vi "Word Search.vi"(8 "error in (no error)":errorcluster, 9 "Solver VI":T1, 10 "Word List":string[](array[string])=["YELLOW", "ORANGE", "PURPLE", "BLUE", "GREEN", "RED"], 11 "Word Search Grid":string[][](array[string])=[["R", "B", "L", "U", "E", "W"], ["E", "G", "N", "A", "R", "O"], ["D", "B", "C", "E", "W", "L"], ["L", "L", "D", "K", "V", "L"], ["P", "U", "R", "P", "L", "E"], ["N", "E", "E", "R", "G", "Y"]]) -> (0 "error out":errorcluster, 2 "All Words Found":bool, 3 "Execution Time":dbl)   [LabVIEW 2024, in "Wordle Scorer.lvlib"]
uses:
  Wordle Scorer.lvlib
  Solver VI Ref Type.ctl
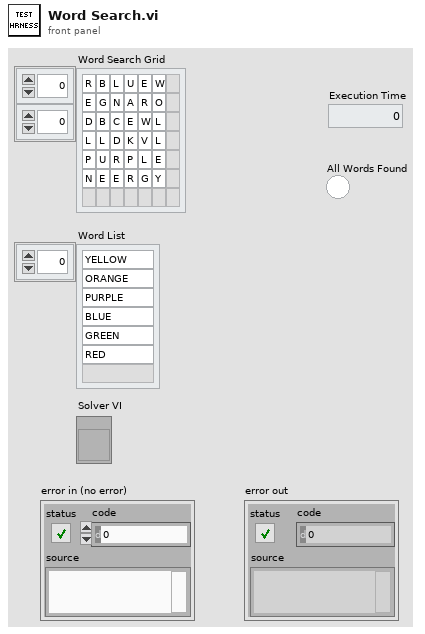
[diagram p1: front panel]
types:
  T1 = typedef "Wordle Scorer.lvlib/Solver VI Ref Type.ctl" = refnum<vi>
  T2 = typedef "Word Search Scorer.lvlib/Solutions--map.ctl" = map{string, T3[]}
  T3 = typedef "Word Search Scorer.lvlib/Letter Index--cluster.ctl" = cluster{"Row":i32, "Column":i32}
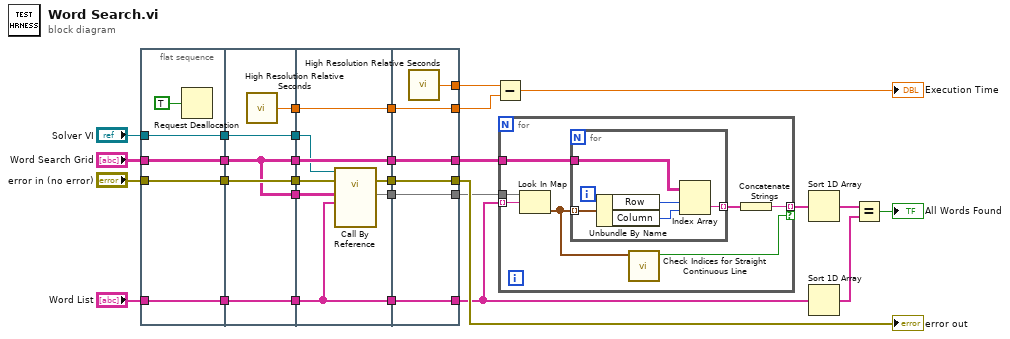
[diagram p0: block diagram]
diagram:
  n1 = flat-sequence {
    tunnel: "error in (no error)" -> [w32]
    tunnel: "Solver VI" -> [w33]
    tunnel: "Word List" -> [w34]
    tunnel: "Word Search Grid" -> [w35]
    tunnel: [w35] -> w4
    tunnel: [w34] -> w3
    tunnel: [w33] -> w2
    tunnel: [w32] -> w1
    tunnel: [w39] -> w29
    tunnel: [w37] -> w28
    tunnel: [w38] -> w26
    tunnel: [w37] -> w22
    tunnel: [w36] -> w21
    tunnel: [w40] -> w7
    tunnel: w4 -> [w37]
    tunnel: w3 -> [w39]
    tunnel: w2 -> [w36]
    tunnel: w1 -> [w40]
    tunnel: w29 -> [w44]
    tunnel: w28 -> [w45]
    tunnel: [w43] -> w27
    tunnel: w26 -> [w48]
    tunnel: [w48] -> w25
    tunnel: [w44] -> w24
    tunnel: [w47] -> w23
    tunnel: w22 -> [w47]
    tunnel: w21 -> [w46]
    tunnel: w7 -> [w42]
    tunnel: [w41] -> w5
    tunnel: w27 -> [w51]
    tunnel: w25 -> [w53]
    tunnel: w24 -> [w50]
    tunnel: w23 -> [w52]
    tunnel: [w54] -> w12
    tunnel: [w53] -> w11
    tunnel: [w52] -> w8
    tunnel: [w51] -> w10
    tunnel: [w50] -> w9
    tunnel: [w49] -> w30
    tunnel: w5 -> [w49]
    frame #0 {
      n2 = Request Deallocation(TRUE ("flag")) -> ()
    }
    frame #1 {
      n3 = call <vilib>:"High Resolution Relative Seconds.vi"() -> ("relative seconds"=w38:dbl)
    }
    frame #2 {
      n4 = call-by-ref "?"(reference=w46, error in=w42, "Word List"=w44, "Word Search Grid"=w45) -> (error out=w41:errorcluster, "Solutions"=w43:T2)  [unwired: 9 in, 1 out]
    }
    frame #3 {
      n5 = call <vilib>:"High Resolution Relative Seconds.vi"() -> ("relative seconds"=w54:dbl)
    }
  }
  n6 = Subtract(x=w12, y=w11) -> (x-y=→"Execution Time":dbl)
  n7 = for {
    tunnel: w9 -> [w60] mode=indexing
    tunnel: w10 -> [w61]
    tunnel: [w58] -> w15 mode=indexing if=w56
    tunnel: w8 -> [w55]
    n8 = Look In Map(map=w61, key=w60) -> (value=w57:T3[])  [unwired: 1 in, 1 out]
    n9 = for {
      tunnel: w57 -> [w66] mode=indexing
      tunnel: [w63] -> w59 mode=indexing
      tunnel: w55 -> [w62]
      n10 = Unbundle By Name(w66) -> ("Row"=w65:i32, "Column"=w64:i32)
      n11 = Index Array(array=w62, index (row)=w65, index (col)=w64) -> (element=w63:string)
    }
    n12 = call "Check Indices for Straight Continuous Line.vi"("Letter Indices"=w57) -> ("Straight Continuous Line?"=w56:bool)  [unwired: 10 in]
    n13 = Concatenate Strings(w59) -> (w58:string)
  }
  n14 = Sort 1D Array(array=w15) -> (sorted array=w16:string[])
  n15 = Sort 1D Array(array=w9) -> (sorted array=w17:string[])
  n16 = Equal?(x=w16, y=w17) -> (x = y?=→"All Words Found":bool)
  "error out" <- w30
